vi "Save Track.vi"(8 "Error In":errorcluster, 9 "Samples Per Channel\\File Size":i32, 10 "Track Name of Copy":string, 11 "Track (File) References":T1) -> (0 "Error Out":errorcluster, 3 "Track (File) References Out":T1)   [LabVIEW 2014]
uses:
  Controls/Track (File) References.ctl
  Controls/Track Enable.ctl
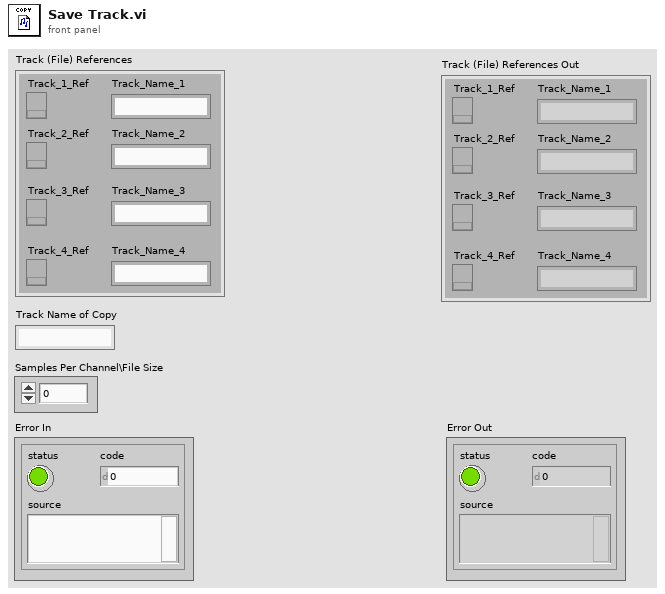
[diagram p1: front panel]
types:
  T1 = typedef "Track (File) References.ctl" = cluster{"Track_1_Ref":refnum<k34>, "Track_2_Ref":refnum<k34>, "Track_3_Ref":refnum<k34>, "Track_4_Ref":refnum<k34>, "Track_Name_1":string, "Track_Name_2":string, "Track_Name_3":string, "Track_Name_4":string}
  T2 = typedef "Track Enable.ctl" = cluster{"Track_0 _Enable ":bool, "Track_1 _Enable ":bool, "Track_2 _Enable ":bool, "Track_3 _Enable ":bool}
  T3 = typedef "4 Track Audio.ctl" = cluster{"Track 0":T4, "Track 1":T4, "Track 2":T4, "Track 3":T4}
  T4 = typedef "Audio In.ctl" = cluster{"AudioIn/Left (N Samples)":i16[], "AudioIn/Right (N Samples)":i16[]}
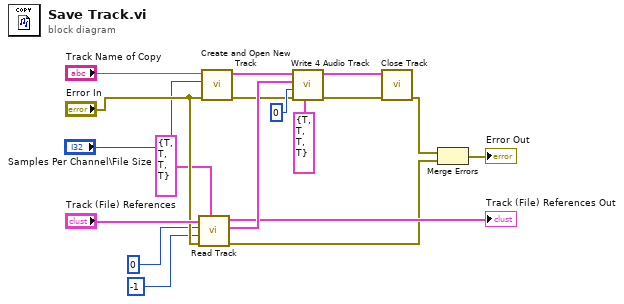
[diagram p0: block diagram]
diagram:
  n1 = call "Read Track.vi"("Track Enable"=T2 {"Track_0 _Enable "=TRUE, "Track_1 _Enable "=TRUE, "Track_2 _Enable "=TRUE, "Track_3 _Enable "=TRUE}, "Error In"="Error In", "Number Of Elements to Read"=i64 -1, "Read Position"=i64 0, "Track (File) References In"="Track (File) References") -> ("Error Out"=w5:errorcluster, "4-Track Audio"=w16:T3, "Track (File) References Out"=→"Track (File) References Out":T1)  [unwired: 4 in]
  n2 = call "Create and Open New Track.vi"("Error In"="Error In", "Samples Per Channel"="Samples Per Channel\\File Size", "Track Name"="Track Name of Copy") -> ("Error Out"=w9:errorcluster, "Track (File) References"=w15:T1)  [unwired: 7 in]
  n3 = call "Write 4 Audio Track.vi"("Track Enable"=T2 {"Track_0 _Enable "=TRUE, "Track_1 _Enable "=TRUE, "Track_2 _Enable "=TRUE, "Track_3 _Enable "=TRUE}, "Error In"=w9, "Write Position"=i64 0, "4-Track Audio"=w16, "Track (File) References In"=w15) -> ("Error Out"=w8:errorcluster, "Track (File) References Out"=w7:T1)  [unwired: 5 in]
  n4 = call "Close Track.vi"("Error In"=w8, "Track (File) References"=w7) -> ("Error Out"=w4:errorcluster)  [unwired: 9 in]
  n5 = Merge Errors(w4, w5) -> (→"Error Out":errorcluster)
